vi "GreaterNoOutput.vi"(0 "A":T1={"Array Num"=[1, 2, 3], "Decimal Index"=0, "stop"=FALSE}, 1 "B":T1={"Array Num"=[1, 2, 3], "Decimal Index"=0, "stop"=FALSE}) -> (3 "Digit Shift":i32, 4 "A Greater":bool, 5 "Equal":bool)   [LabVIEW 2025]
doc: "Doesn't work with sign of numbers yet."
uses:
  Number.ctl
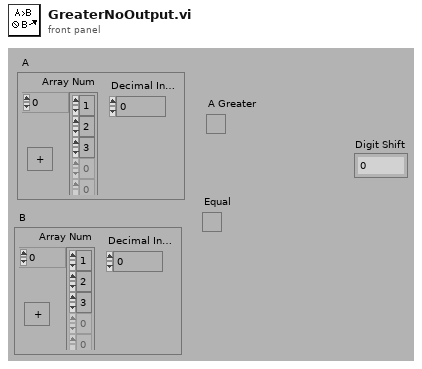
[diagram p1: front panel]
types:
  T1 = typedef "Number.ctl" = cluster{"Array Num":i8[], "Decimal Index":i32, "stop":bool}
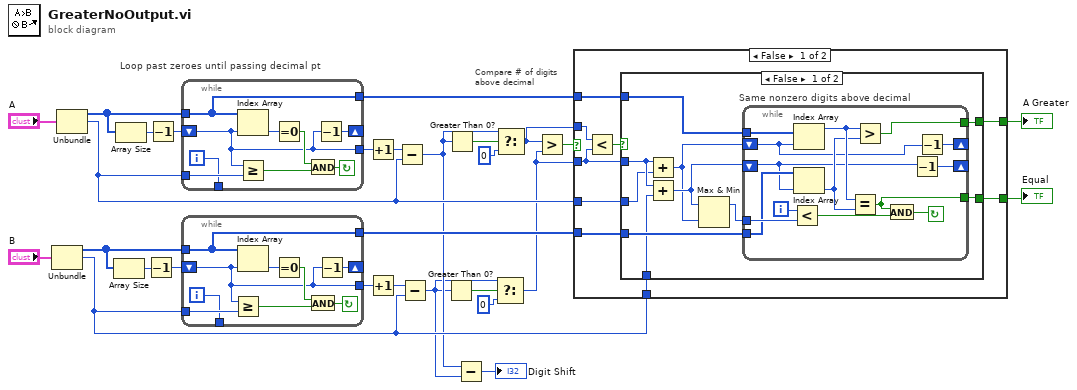
[diagram p0: block diagram]
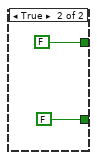
[diagram p2: hidden frame]
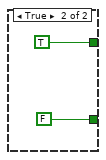
[diagram p3: hidden frame]
diagram:
  # "Compare # of digits above decimal"
  # "Loop past zeroes until passing decimal pt"
  n1 = Unbundle("B") -> ("Array Num"=w20:i8[], "Decimal Index"=w13:i32)  [unwired: 1 out]
  n2 = Unbundle("A") -> ("Array Num"=w21:i8[], "Decimal Index"=w14:i32)  [unwired: 1 out]
  n3 = Array Size(array=w20) -> (size(s)=w25:i32)
  n4 = Array Size(array=w21) -> (size(s)=w23:i32)
  n5 = Decrement(x=w25) -> (x-1=w4:i32)
  n6 = Decrement(x=w23) -> (x-1=w5:i32)
  n7 = while {
    tunnel: [w34] -> w27
    tunnel: [w30] -> w22
    tunnel: w21 -> [w34]
    tunnel: w14 -> [w33]
    shift-right: [w31] -> _
    shift-left: w5 -> [w30]
    tunnel: [w29] -> _
    i -> [w29]
    stop <- w37 continue-if-true
    n8 = Index Array(array=w34, index=w30) -> (element=w36:i8)
    n9 = Greater Or Equal?(x=w30, y=w33) -> (x >= y?=w35:bool)
    n10 = Equal To 0?(x=w36) -> (x = 0?=w32:bool)
    n11 = And(x=w32, y=w35) -> (x .and. y?=w37:bool)
    n12 = Decrement(x=w30) -> (x-1=w31:i32)
  }
  n13 = while {
    tunnel: [w44] -> w26
    tunnel: [w39] -> w24
    tunnel: w20 -> [w44]
    tunnel: w13 -> [w42]
    shift-right: [w40] -> _
    shift-left: w4 -> [w39]
    tunnel: [w38] -> _
    i -> [w38]
    stop <- w46 continue-if-true
    n14 = Greater Or Equal?(x=w39, y=w42) -> (x >= y?=w43:bool)
    n15 = Index Array(array=w44, index=w39) -> (element=w45:i8)
    n16 = Equal To 0?(x=w45) -> (x = 0?=w41:bool)
    n17 = And(x=w41, y=w43) -> (x .and. y?=w46:bool)
    n18 = Decrement(x=w39) -> (x-1=w40:i32)
  }
  n19 = Increment(x=w22) -> (x+1=w16:i32)
  n20 = Increment(x=w24) -> (x+1=w15:i32)
  n21 = Subtract(x=w16, y=w14) -> (x-y=w3:i32)
  n22 = Subtract(x=w15, y=w13) -> (x-y=w2:i32)
  n23 = Greater Than 0?(x=w2) -> (x > 0?=w8:bool)
  n24 = Greater Than 0?(x=w3) -> (x > 0?=w9:bool)
  n25 = Subtract(x=w3, y=w2) -> (x-y=→"Digit Shift":i32)
  n26 = Select(t=w2, s=w8, f=0) -> (s? t:f=w6:i32)
  n27 = Select(t=w3, s=w9, f=0) -> (s? t:f=w10:i32)
  n28 = Greater?(x=w10, y=w6) -> (0:w28:bool)
  n29 = case shown="False" w28 {
    tunnel: [w54 TRUE] -> w12
    tunnel: w26 -> [w53 _]
    tunnel: w6 -> [w48 _]
    tunnel: w10 -> [w47 _]
    tunnel: w27 -> [w52 _]
    tunnel: [w51 FALSE] -> w17
    tunnel: w14 -> [w50 _]
    tunnel: w13 -> [w49 _]
    frame False {
      n30 = Less?(x=w47, y=w48) -> (x < y?=w55:bool)
      n31 = case shown="False" w55 {
        tunnel: [w63 FALSE] -> w54
        tunnel: w53 -> [w64 _]
        tunnel: w52 -> [w65 _]
        tunnel: [w59 FALSE] -> w51
        tunnel: w50 -> [w61 _]
        tunnel: w49 -> [w60 _]
        tunnel: w48 -> [w62 _]
        frame False {
          # "Same nonzero digits above decimal"
          n32 = Add(x=w62, y=w61) -> (x+y=w56:i32)
          n33 = Add(x=w62, y=w60) -> (x+y=w57:i32)
          n34 = Max & Min(x=w57, y=w56) -> (max(x,y)=w58:i32)  [unwired: 1 out]
          n35 = while {
            tunnel: w58 -> [w73]
            tunnel: [w74] -> w59
            tunnel: [w75] -> w63
            tunnel: w64 -> [w70]
            tunnel: w65 -> [w71]
            shift-right: [w68] -> _
            shift-left: w56 -> [w66]
            shift-right: [w69] -> _
            shift-left: w57 -> [w67]
            i -> [w72]
            stop <- w78 continue-if-true
            n36 = Less?(x=w72, y=w73) -> (x < y?=w79:bool)
            n37 = Index Array(array=w71, index=w66) -> (element=w77:i8)
            n38 = Index Array(array=w70, index=w67) -> (element=w76:i8)
            n39 = Equal?(x=w77, y=w76) -> (x = y?=w74:bool)
            n40 = Greater?(x=w77, y=w76) -> (0:w75:bool)
            n41 = And(x=w74, y=w79) -> (x .and. y?=w78:bool)
            n42 = Decrement(x=w67) -> (x-1=w69:i32)
            n43 = Decrement(x=w66) -> (x-1=w68:i32)
          }
        }
        frame True {
        }
      }
    }
    frame True {
    }
  }
  "A Greater" <- w12
  "Equal" <- w17
